vi "debug.vi"   [LabVIEW 2010, in "LASA Beta.lvrbt"]
uses:
  LASA Beta.lvrbt
  <vilib>/NXT/Block Support/NXT_ButtonSelector.ctl
  <vilib>/NXT/Subs/LVHSConnector.ctl
  <vilib>/NXT/NXTIO Xnodes/AddressXNode/NXTIOAddress.xnode
  <vilib>/NXT/Subs/MotorXNode.Servo Type.ctl
  <vilib>/NXT/Subs/MotorXNode.1Servo.ctl
  <vilib>/NXT/NXTIO Xnodes/NXTIOXNode/NXTIO.xnode
  <vilib>/NXT/Dual Mode Library/Display/clearDisplay.vi
  <vilib>/NXT/Dual Mode Library/Display/drawText.vi
  <vilib>/NXT/Dual Mode Library/Sensors/readNXTButton.vi
  op_run.vi
  <vilib>/NXT/NXTIO Xnodes/NXTIONodeSubVIs/TETRIX IO Move Servos.vi
types:
  T1 = typedef "LVHSConnector.ctl" = cluster{"Hardware":string, "Flattened String":string}
  T2 = typedef "NXT_ButtonSelector.ctl" = u16
  T3 = typedef "MotorXNode.Servo Type.ctl" = enum16{"Servo"}
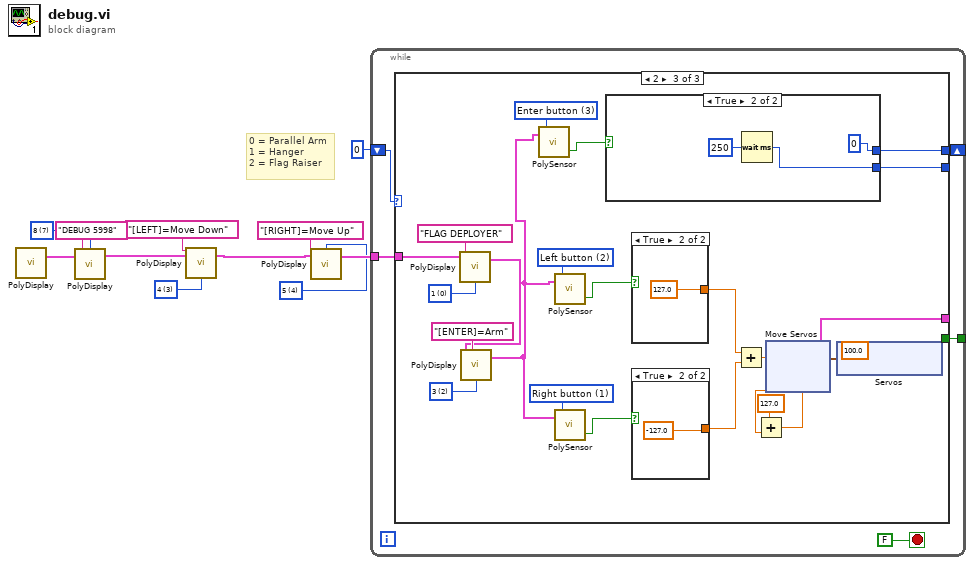
[diagram p0: block diagram]
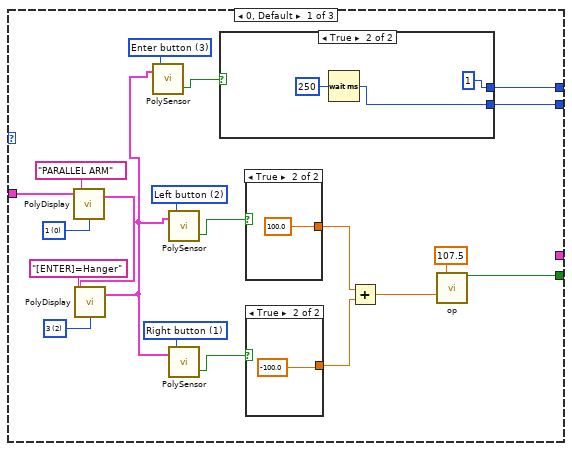
[diagram p2: hidden frame]
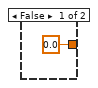
[diagram p3: hidden frame]
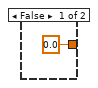
[diagram p4: hidden frame]
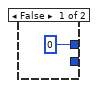
[diagram p5: hidden frame]
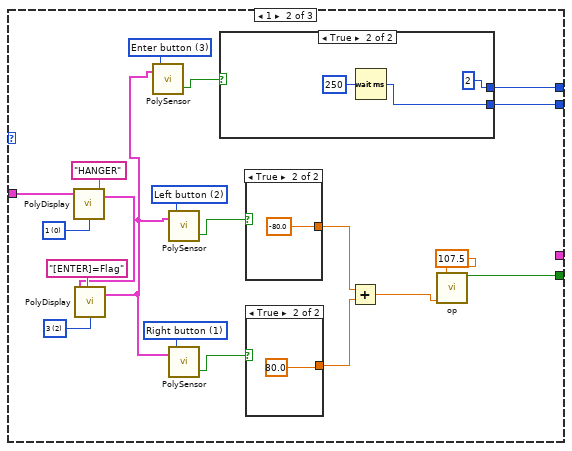
[diagram p6: hidden frame]
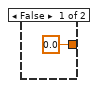
[diagram p7: hidden frame]
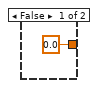
[diagram p8: hidden frame]
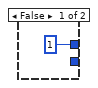
[diagram p9: hidden frame]
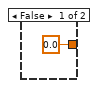
[diagram p10: hidden frame]
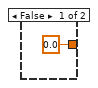
[diagram p11: hidden frame]
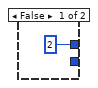
[diagram p12: hidden frame]
diagram:
  w1 = i16 4 items=["1", "2", "3", "4", "5", "6", "7", "8"] ("Line")
  w7 = i16 3 items=["1", "2", "3", "4", "5", "6", "7", "8"] ("Line")
  w9 = i16 7 items=["1", "2", "3", "4", "5", "6", "7", "8"] ("Line")
  # "0 = Parallel Arm\n1 = Hanger\n2 = Flag Raiser"
  n1 = call-poly <vilib>:"PolyDisplay.vi"() -> ("NXT"=w11:T1)  [unwired: 4 in]
  n2 = call-poly <vilib>:"PolyDisplay.vi"("Text"="DEBUG 5998", "NXT"=w11, "Line"=w9) -> ("NXT"=w5:T1)  [unwired: 1 in]
  n3 = call-poly <vilib>:"PolyDisplay.vi"("Text"="[LEFT]=Move Down", "NXT"=w5, "Line"=w7) -> ("NXT"=w3:T1)  [unwired: 1 in]
  n4 = call-poly <vilib>:"PolyDisplay.vi"("Text"="[RIGHT]=Move Up", "NXT"=w3, "Line"=w1) -> ("NXT"=w2:T1)  [unwired: 1 in]
  n5 = while {
    shift-right: [w13] -> _
    shift-left: 0 -> [w15]
    tunnel: w2 -> [w14]
    tunnel: [w12] -> _
    stop <- FALSE stop-if-true
    n6 = case shown="2" w15 {
      tunnel: w14 -> [w20 w48 w80]
      tunnel: [w29 w57 w87] -> w13
      tunnel: [w24 w52 _] -> w12
      tunnel: [w19 w47 w79] -> _
      tunnel: [_ _ w76] -> _
      frame 0, Default {
        w26 = T2 1 items=["Enter button"=3, "Left button"=2, "Right button"=1] ("Button (Enter button)")
        w28 = T2 2 items=["Enter button"=3, "Left button"=2, "Right button"=1] ("Button (Enter button)")
        w31 = i16 2 items=["1", "2", "3", "4", "5", "6", "7", "8"] ("Line")
        w34 = i16 0 items=["1", "2", "3", "4", "5", "6", "7", "8"] ("Line")
        w36 = T2 3 items=["Enter button"=3, "Left button"=2, "Right button"=1] ("Button (Enter button)")
        n7 = call-poly <vilib>:"PolyDisplay.vi"("Text"="PARALLEL ARM", "NXT"=w20, "Line"=w34) -> ("NXT"=w30:T1)  [unwired: 1 in]
        n8 = call-poly <vilib>:"PolyDisplay.vi"("Text"="[ENTER]=Hanger", "NXT"=w30, "Line"=w31) -> ("NXT"=w18:T1)  [unwired: 1 in]
        n9 = call-poly <vilib>:"PolySensor.vi"("Button (Enter button)"=w36, "NXT"=w18) -> ("Yes/No"=w33:bool)  [unwired: 1 in, 1 out]
        n10 = call-poly <vilib>:"PolySensor.vi"("Button (Enter button)"=w28, "NXT"=w18) -> ("Yes/No"=w27:bool)  [unwired: 1 in, 1 out]
        n11 = call-poly <vilib>:"PolySensor.vi"("Button (Enter button)"=w26, "NXT"=w18) -> ("Yes/No"=w25:bool)  [unwired: 1 in, 1 out]
        n12 = case shown="True" w33 {
          tunnel: [0 1] -> w29
          tunnel: [_ w42] -> w19
          frame False {
          }
          frame True {
            n13 = Wait (ms)(milliseconds to wait=u32 250) -> (millisecond timer value=w42:u32)
          }
        }
        n14 = case shown="True" w27 {
          tunnel: [0.0 ("Left Drive") 100.0 ("Left Drive")] -> w23
          frame False {
          }
          frame True {
          }
        }
        n15 = case shown="True" w25 {
          tunnel: [0.0 ("Left Drive") -100.0 ("Left Drive")] -> w22
          frame False {
          }
          frame True {
          }
        }
        n16 = Add(x=w23, y=w22) -> (x+y=w21:dbl)
        n17 = call-poly "op.vi"("Dump Control"=107.5, "Arm Control"=w21) -> ("Chain OUT"=w24:bool)  [unwired: 13 in]
      }
      frame 1 {
        w54 = T2 1 items=["Enter button"=3, "Left button"=2, "Right button"=1] ("Button (Enter button)")
        w56 = T2 2 items=["Enter button"=3, "Left button"=2, "Right button"=1] ("Button (Enter button)")
        w59 = i16 2 items=["1", "2", "3", "4", "5", "6", "7", "8"] ("Line")
        w62 = i16 0 items=["1", "2", "3", "4", "5", "6", "7", "8"] ("Line")
        w64 = T2 3 items=["Enter button"=3, "Left button"=2, "Right button"=1] ("Button (Enter button)")
        n18 = call-poly <vilib>:"PolyDisplay.vi"("Text"="HANGER", "NXT"=w48, "Line"=w62) -> ("NXT"=w58:T1)  [unwired: 1 in]
        n19 = call-poly <vilib>:"PolyDisplay.vi"("Text"="[ENTER]=Flag", "NXT"=w58, "Line"=w59) -> ("NXT"=w46:T1)  [unwired: 1 in]
        n20 = call-poly <vilib>:"PolySensor.vi"("Button (Enter button)"=w64, "NXT"=w46) -> ("Yes/No"=w61:bool)  [unwired: 1 in, 1 out]
        n21 = call-poly <vilib>:"PolySensor.vi"("Button (Enter button)"=w56, "NXT"=w46) -> ("Yes/No"=w55:bool)  [unwired: 1 in, 1 out]
        n22 = call-poly <vilib>:"PolySensor.vi"("Button (Enter button)"=w54, "NXT"=w46) -> ("Yes/No"=w53:bool)  [unwired: 1 in, 1 out]
        n23 = case shown="True" w61 {
          tunnel: [1 2] -> w57
          tunnel: [_ w70] -> w47
          frame False {
          }
          frame True {
            n24 = Wait (ms)(milliseconds to wait=u32 250) -> (millisecond timer value=w70:u32)
          }
        }
        n25 = case shown="True" w55 {
          tunnel: [0.0 ("Left Drive") -80.0 ("Left Drive")] -> w51
          frame False {
          }
          frame True {
          }
        }
        n26 = case shown="True" w53 {
          tunnel: [0.0 ("Left Drive") 80.0 ("Left Drive")] -> w50
          frame False {
          }
          frame True {
          }
        }
        n27 = Add(x=w51, y=w50) -> (x+y=w49:dbl)
        n28 = call-poly "op.vi"("Dump Control"=107.5, "Lift String Control"=w49) -> ("Chain OUT"=w52:bool)  [unwired: 13 in]
      }
      frame 2 {
        (unwired) 100.0 ("t")
        w84 = T2 1 items=["Enter button"=3, "Left button"=2, "Right button"=1] ("Button (Enter button)")
        w86 = T2 2 items=["Enter button"=3, "Left button"=2, "Right button"=1] ("Button (Enter button)")
        w89 = i16 2 items=["1", "2", "3", "4", "5", "6", "7", "8"] ("Line")
        w92 = i16 0 items=["1", "2", "3", "4", "5", "6", "7", "8"] ("Line")
        w94 = T2 3 items=["Enter button"=3, "Left button"=2, "Right button"=1] ("Button (Enter button)")
        n29 = call-poly <vilib>:"PolyDisplay.vi"("Text"="FLAG DEPLOYER", "NXT"=w80, "Line"=w92) -> ("NXT"=w88:T1)  [unwired: 1 in]
        n30 = call-poly <vilib>:"PolyDisplay.vi"("Text"="[ENTER]=Arm", "NXT"=w88, "Line"=w89) -> ("NXT"=w78:T1)  [unwired: 1 in]
        n31 = call-poly <vilib>:"PolySensor.vi"("Button (Enter button)"=w94, "NXT"=w78) -> ("Yes/No"=w91:bool)  [unwired: 1 in, 1 out]
        n32 = call-poly <vilib>:"PolySensor.vi"("Button (Enter button)"=w86, "NXT"=w78) -> ("Yes/No"=w85:bool)  [unwired: 1 in, 1 out]
        n33 = call-poly <vilib>:"PolySensor.vi"("Button (Enter button)"=w84, "NXT"=w78) -> ("Yes/No"=w83:bool)  [unwired: 1 in, 1 out]
        n34 = case shown="True" w91 {
          tunnel: [2 0] -> w87
          tunnel: [_ w109] -> w79
          frame False {
          }
          frame True {
            n35 = Wait (ms)(milliseconds to wait=u32 250) -> (millisecond timer value=w109:u32)
          }
        }
        n36 = case shown="True" w85 {
          tunnel: [0.0 ("Left Drive") 127.0 ("Left Drive")] -> w82
          frame False {
          }
          frame True {
          }
        }
        n37 = case shown="True" w83 {
          tunnel: [0.0 ("Left Drive") -127.0 ("Left Drive")] -> w81
          frame False {
          }
          frame True {
          }
        }
        n38 = Add(x=w82, y=w81) -> (x+y=w74:dbl)
        n39 = Add(x=127.0, y=w74) -> (x+y=w73:dbl)
        n40 = xnode "Servos"() -> ("Servo"=w77:cluster{"Servo":T3, "Address":i16})
        n41 = xnode "Move Servos"("Position 1"=w73, "Servos"=w77) -> ("NXT"=w76:T1)  [unwired: 1 in]
      }
    }
  }
